vi "Negate (single).vi"(8 "error in (no error)":errorcluster, 11 "XY-data":cluster{"X-array":dbl[], "Y-array":dbl[]} {"Y-array" format="%.2p"; "X-array" format="%.2p"}) -> (0 "error out":errorcluster, 3 "XY-data out":cluster{"X-array":dbl[], "Y-array":dbl[]} {"Y-array" format="%.2p"; "X-array" format="%.2p"})   [LabVIEW 2019, in "xy_utilities.lvlib"]
doc: "Negates <b>XY-data</b>'s y array.\n\nWire data to the data input to determine the polymorphic instance to use or manually select the instance."
uses:
  xy_utilities.lvlib
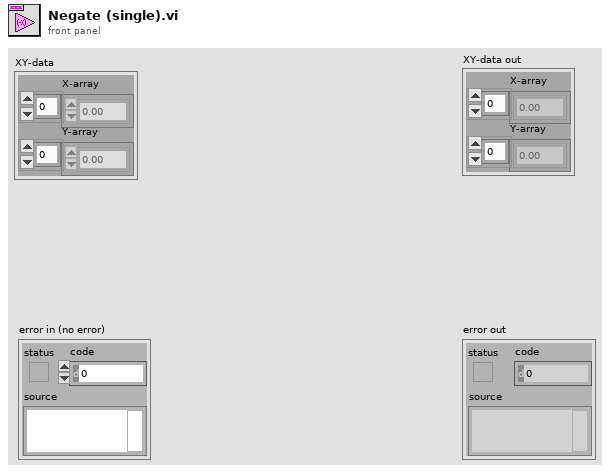
[diagram p1: front panel]
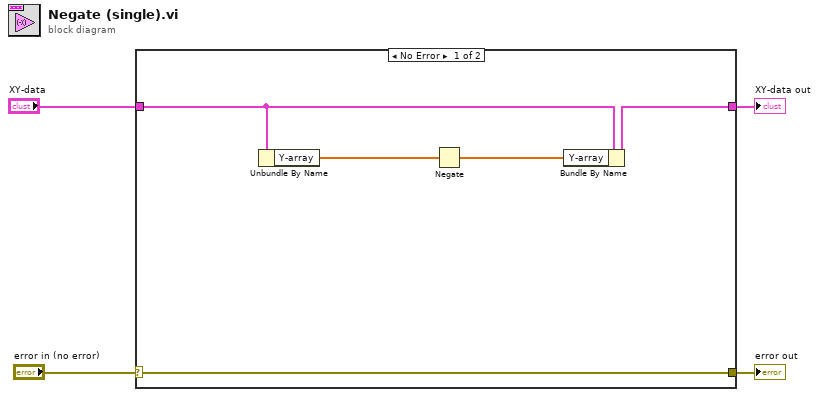
[diagram p0: block diagram]
diagram:
  n1 = case shown="No Error" "error in (no error)" {
    selector: "error in (no error)" -> [w9 w11]
    tunnel: [w9 w11] -> w3
    tunnel: "XY-data" -> [w8 w10]
    tunnel: [w7 w10] -> w1
    frame No Error {
      n2 = Unbundle By Name(w8) -> ("Y-array"=w6:dbl[])
      n3 = Negate(x=w6) -> (-x=w5:dbl[])
      n4 = Bundle By Name(cluster=w8, "Y-array"=w5) -> (w7:cluster{"X-array":dbl[], "Y-array":dbl[]})
    }
    frame Error {
    }
  }
  "error out" <- w3
  "XY-data out" <- w1
